vi "Read Geometry Definition Double.vi"(8 "error in":errorcluster, 9 "Feature":string, 10 "Part Type":T1, 11 "Config Manager in":refnum<class "Config Manager Class.lvclass">) -> (0 "error out":errorcluster, 2 "Geometry Definition":dbl, 3 "Config Manager out":refnum<class "Config Manager Class.lvclass">)   [LabVIEW 2011, in "Config Manager Class.lvclass"]
uses:
  Config Manager Class.lvclass
  Type Definitions/Part Type.ctl
  Config Manager Class.lvclass/Config Manager Class.ctl
  <vilib>/Utility/config.llb/Read Key (Double).vi
  <vilib>/Utility/config.llb/NI_LVConfig.lvlib
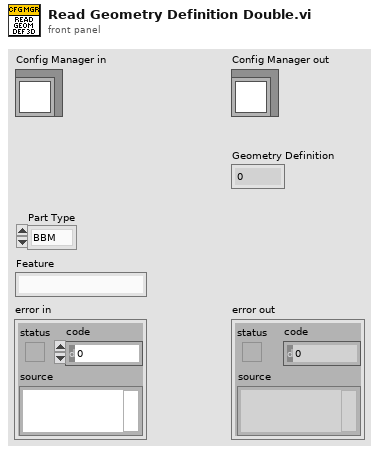
[diagram p1: front panel]
types:
  T1 = typedef "Part Type.ctl" = enum16{"BBM", "HDI"}
  T2 = typedef "NI_LVConfig.lvlib/Config Data RefNum.ctl" = refnum<k1>
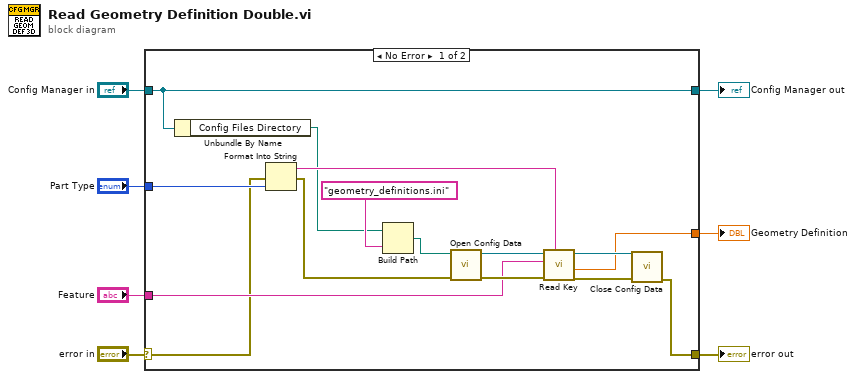
[diagram p0: block diagram]
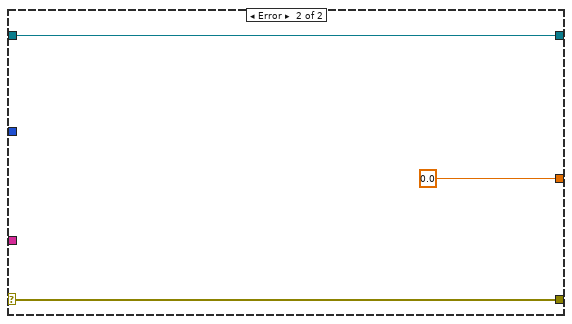
[diagram p2: hidden frame]
diagram:
  n1 = case shown="No Error" "error in" {
    selector: "error in" -> [w11 w25]
    tunnel: [w12 w25] -> w6
    tunnel: [w15 w24] -> w4
    tunnel: "Config Manager in" -> [w15 w24]
    tunnel: "Part Type" -> [w17 _]
    tunnel: "Feature" -> [w13 _]
    tunnel: [w8 0.0 ("value")] -> w1
    frame No Error {
      n2 = Unbundle By Name(w15) -> ("Config Files Directory"=w14:path)
      n3 = Format Into String(error in=w11, w17) -> (resulting string=w16:string, error out=w10:errorcluster)  [unwired: 2 in]
      n4 = Build Path(base path=w14, name or relative path="geometry_definitions.ini") -> (appended path=w21:path)
      n5 = call <vilib>:"Open Config Data.vi"("error in (no error)"=w10, "configuration file path"=w21) -> ("error out"=w19:errorcluster, "refnum"=w20:T2)  [unwired: 7 in, 1 out]
      n6 = call-poly <vilib>:"Read Key.vi"("section"=w16, "error in (no error)"=w19, "key"=w13, "refnum"=w20) -> ("error out"=w9:errorcluster, "value"=w8:dbl, "refnum out"=w18:T2)  [unwired: 4 in, 1 out]
      n7 = call <vilib>:"Close Config Data.vi"("error in (no error)"=w9, "refnum"=w18) -> ("error out"=w12:errorcluster)  [unwired: 8 in, 1 out]
    }
    frame Error {
    }
  }
  "error out" <- w6
  "Config Manager out" <- w4
  "Geometry Definition" <- w1
